vi "FP_Size VI to Deoration.vi"(8 "Error":errorcluster, 9 "FPSet":T2={"Menu Bar"=FALSE, "Position"=enum."MID-CTR", "Decoration index"=0, "border(px)"=-2, "Monitor #"=0}, 11 "VI Ref":refnum<vi>) -> (0 "Error Out":errorcluster, 3 "VI Ref Out":refnum<vi>)   [LabVIEW 2017]
doc: "sets up a fp to center of monitor 1 around largest decoration. shows scroll bars if developing and hides them if not."
uses:
  FP_Size VI to Decoration Simple.vi/TypeDefs_Utility/Cluster_FP Set.ctl
  FP_Size VI to Decoration Simple.vi/TypeDefs_Utility/ENUM RB_Pos_Quadrant Position.ctl
  <vilib>/Utility/miscctls.llb/LVAllMonitorsDisplayTypeDef.ctl
  FP_Size VI to Decoration Simple.vi/TypeDefs_Utility/Cluster_Pos_Top Left position.ctl
panel:
  out "Display:All Monitors":T1
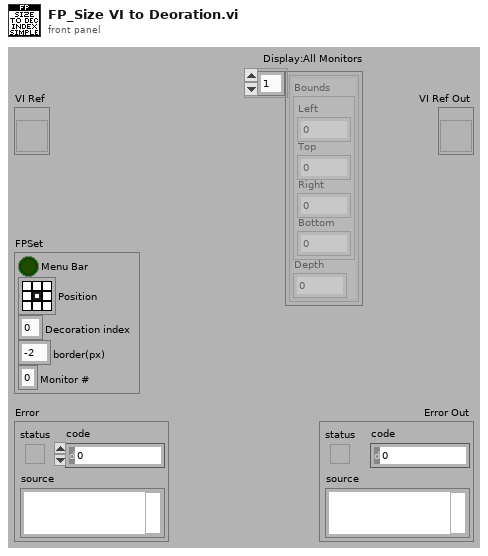
[diagram p1: front panel]
types:
  T1 = typedef "LVAllMonitorsDisplayTypeDef.ctl" = cluster{"Bounds":cluster{"Left":i16, "Top":i16, "Right":i16, "Bottom":i16}, "Depth":i16}[]
  T2 = typedef "Cluster_FP Set.ctl" = cluster{"Menu Bar":bool, "Position":T3, "Decoration index":i32, "border(px)":i32, "Monitor #":i32}
  T3 = typedef "ENUM RB_Pos_Quadrant Position.ctl" = enum32{"LFT-TOP", "MID-TOP", "RGT-TOP", "LFT-CTR", "MID-CTR", "RGT-CTR", "LFT-BOT", "MID-BOT", "RGT-BOT"}
  T4 = typedef "Cluster_Pos_Top Left position.ctl" = cluster{"Left":i16, "Top":i16}
  T5 = enum32{"Invalid", "Standard", "Closed", "Hidden", "Minimized", "Maximized"}
  T6 = cluster{"Bounds":cluster{"Left":i16, "Top":i16, "Right":i16, "Bottom":i16}, "Depth":i16}
  T7 = cluster{"Left":i16, "Top":i16, "Right":i16, "Bottom":i16}
  T8 = typedef "LVRectTypeDef.ctl" = cluster{"Left":i16, "Top":i16, "Right":i16, "Bottom":i16}
  T9 = typedef "LVPositionTypeDef.ctl" = cluster{"Left":i32, "Top":i32}
  T10 = typedef "LVBoundsTypeDef.ctl" = cluster{"Width":u32, "Height":u32}
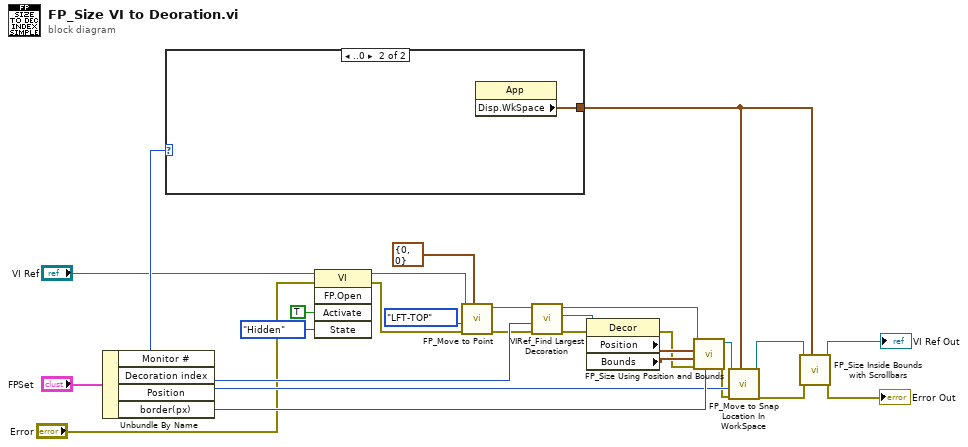
[diagram p0: block diagram]
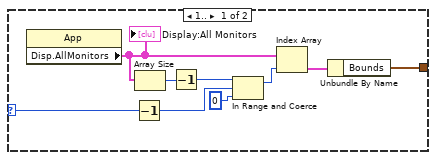
[diagram p2: hidden frame]
diagram:
  n1 = Unbundle By Name("FPSet") -> ("Monitor #"=w27:i32, "Decoration index"=w20:i32, "Position"=w14:T3, "border(px)"=w15:i32)
  n2 = case shown="..0" w27 {
    selector: w27 -> [w34 _]
    tunnel: [w29 w38] -> w2
    frame 1.. {
      n3 = property class="App"() -> ("Disp.AllMonitors"=w32:T1)  [unwired: 2 in, 2 out]
      "Display:All Monitors" <- w32
      n4 = Decrement(x=w34) -> (x-1=w33:i32)
      n5 = Array Size(array=w32) -> (size(s)=w37:i32)
      n6 = Decrement(x=w37) -> (x-1=w36:i32)
      n7 = In Range and Coerce(upper limit=w36, x=w33, lower limit=0) -> (coerced(x)=w31:i32)  [unwired: 1 out]
      n8 = Index Array(array=w32, index=w31) -> (element=w30:T6)
      n9 = Unbundle By Name(w30) -> ("Bounds"=w29:T7)
    }
    frame ..0 {
      n10 = property class="App"() -> ("Disp.WkSpace"=w38:T8)  [unwired: 2 in, 2 out]
    }
  }
  n11 = invoke class="VI" method="FP.Open"(reference="VI Ref", error in="Error", "Activate"=TRUE ("Activate?"), "State"=T5."Hidden") -> (reference out=w22:refnum<vi>, error out=w11:errorcluster)  [unwired: 1 in, 3 out]
  n12 = call "FP_Move to Point.vi"("Target Point"=T4 {"Left"=0, "Top"=0}, "Error"=w11, "FP Position"=ENUM_RB_Pos_Quadrant_Position."LFT-TOP", "VI"=w22) -> ("Error Out"=w13:errorcluster, "VI Out"=w21:refnum<vi>)  [unwired: 6 in]
  n13 = call "VIRef_Find Largest Decoration.vi"("Error"=w13, "Decoration index"=w20, "VI's Ref"=w21) -> ("Error Out"=w9:errorcluster, "Decor Refnum Out"=w19:refnum<vi>, "Calling VI's Ref Out"=w16:refnum<vi>)  [unwired: 2 in, 4 out]
  n14 = property class="Decor"(reference=w19, error in=w9) -> (error out=w10:errorcluster, "Position"=w18:T9, "Bounds"=w17:T10)  [unwired: 1 out]
  n15 = call "FP_Size Using Position and Bounds.vi"("Border Spacing"=w15, "Error"=w10, "Bounds"=w17, "Position"=w18, "VI"=w16) -> ("Error Out"=w7:errorcluster, "VI Out"=w8:refnum<vi>)  [unwired: 4 in, 1 out]
  n16 = call "FP_Move to Snap Location In WorkSpace.vi"("WkSpace"=w2, "Error"=w7, "Snap Location"=w14, "VI"=w8) -> ("Error Out"=w6:errorcluster, "VI Out"=w4:refnum<vi>)  [unwired: 6 in]
  n17 = call "FP_Size Inside Bounds with Scrollbars.vi"("WkSpace"=w2, "Error"=w6, "VI"=w4) -> ("Error Out"=→"Error Out":errorcluster, "VI Out"=→"VI Ref Out":refnum<vi>)  [unwired: 6 in, 1 out]
